vi "can be index.vi"(8 "error in (no error)":errorcluster, 9 "string":string, 11 "JSON Value in":refnum<class "JSON Value.lvclass">) -> (0 "error out":errorcluster, 1 "index":i32, 2 "last value?":bool, 3 "valid index?":bool)   [LabVIEW 2016, in "JSON Value.lvclass"]
uses:
  JSON Value.lvclass
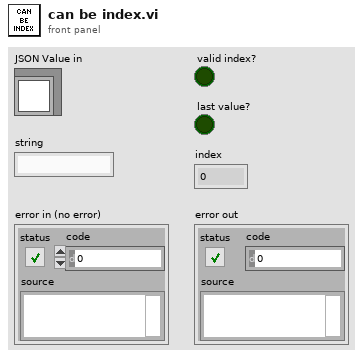
[diagram p1: front panel]
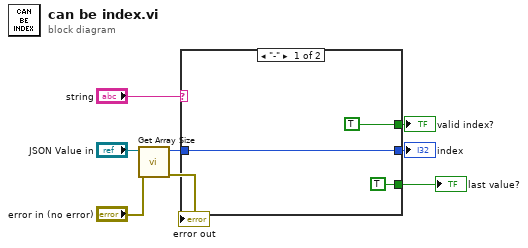
[diagram p0: block diagram]
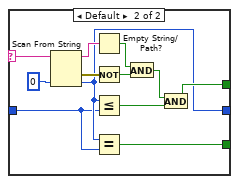
[diagram p2: hidden frame]
diagram:
  n1 = call "Get Array Size.vi"("error in (no error)"="error in (no error)", "JSON Value in"="JSON Value in") -> ("error out"=→"error out":errorcluster, "size(s)"=w4:i32)  [unwired: 8 in]
  n2 = case shown="\"-\"" "string" {
    selector: "string" -> [_ w19]
    tunnel: [TRUE w15] -> w7
    tunnel: [w10 w14] -> w6
    tunnel: w4 -> [w10 w13]
    tunnel: [TRUE w12] -> w2
    frame "-" {
    }
    frame Default {
      n3 = Scan From String(input string=w19, default 1=0 ("value")) -> (remaining string=w20:string, error out=w21:errorcluster, output 1=w14:i32)  [unwired: 3 in, 1 out]
      n4 = Empty String/Path?(string/path=w20) -> (empty?=w23:bool)
      n5 = Not(x=w21) -> (.not. x?=w22:bool)
      n6 = Less Or Equal?(x=w14, y=w13) -> (x <= y?=w16:bool)
      n7 = Equal?(x=w14, y=w13) -> (x = y?=w12:bool)
      n8 = And(x=w23, y=w22) -> (x .and. y?=w17:bool)
      n9 = And(x=w17, y=w16) -> (x .and. y?=w15:bool)
    }
  }
  "valid index?" <- w7
  "index" <- w6
  "last value?" <- w2
